vi "10bwrite.vi"() -> ()   [LabVIEW 2013]
panel:
  in  "text":string
  in  "file path (use dialog)":path
  # "G.SURESH\n23A91A0417\nECE-A"
  # "10B) FILE I/O OPERATIONS (WRITE OPERATION)"
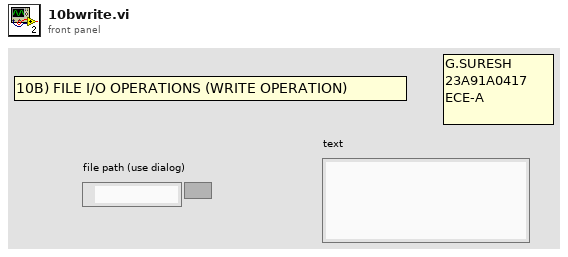
[diagram p1: front panel]
types:
  T1 = enum16{"open", "replace", "create", "open or create", "replace or create", "replace or create with confirmation"}
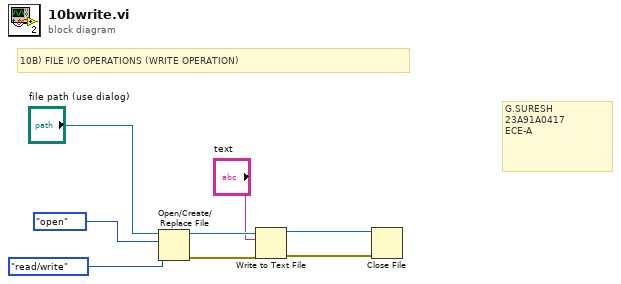
[diagram p0: block diagram]
diagram:
  # "G.SURESH\n23A91A0417\nECE-A"
  # "10B) FILE I/O OPERATIONS (WRITE OPERATION)"
  n1 = Open/Create/Replace File(file path (use dialog)="file path (use dialog)", operation (0:open)=T1."open", access (0:read/write)=enum16{"read/write", "read-only", "write-only"}."read/write") -> (refnum out=w8:refnum<file>, error out=w6:errorcluster)  [unwired: 3 in, 1 out]
  n2 = Write to Text File(file (use dialog)=w8, text="text", error in=w6) -> (refnum out=w7:refnum<file>, error out=w5:errorcluster)  [unwired: 1 in, 1 out]
  n3 = Close File(refnum=w7, error in=w5) -> ()  [unwired: 2 out]
